vi "HumanExecute.vi"(8 "error in (no error)":errorcluster) -> (0 "error out":errorcluster)   [LabVIEW 2020]
doc: "Execute for Human\n\ninput:\n error in (cluster)\n\noutput:\n error out (cluster)"
uses:
  <vilib>/Rock Robotics/WPI/Joystick/XBox Buttons Indexer.ctl
  <vilib>/Rock Robotics/WPI/Joystick/XBox Axes Indexer.ctl
  Arm/ArmGamePiecePreset.ctl
  Arm/ArmPositionPreset.ctl
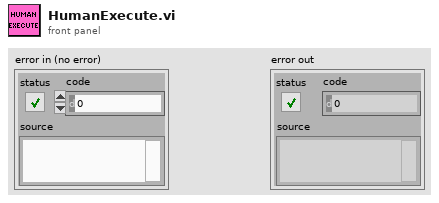
[diagram p1: front panel]
types:
  T1 = typedef "XBox Buttons Indexer.ctl" = enum16{"A", "B", "X", "Y", "Left Bumper", "Right Bumper", "Back", "Start", "Left Joystick", "Right Joystick"}
  T2 = typedef "XBox Axes Indexer.ctl" = enum16{"Left X", "Left Y", "Left Trigger", "Right Trigger", "Right X", "Right Y"}
  T3 = typedef "WPI_JoystickDevRef.ctl" = cluster{"Device":T4}
  T4 = typedef "WPI_JoystickDeviceEnum.ctl" = enum16{"USB 0", "USB 1", "USB 2", "USB 3", "USB 4", "USB 5"}
  T5 = typedef "ArmGamePiecePreset.ctl" = enum16{"Cube", "Cone"}
  T6 = typedef "ArmPositionPreset.ctl" = enum16{"Upper", "Lower", "Middle", "Shelf", "Floor"}
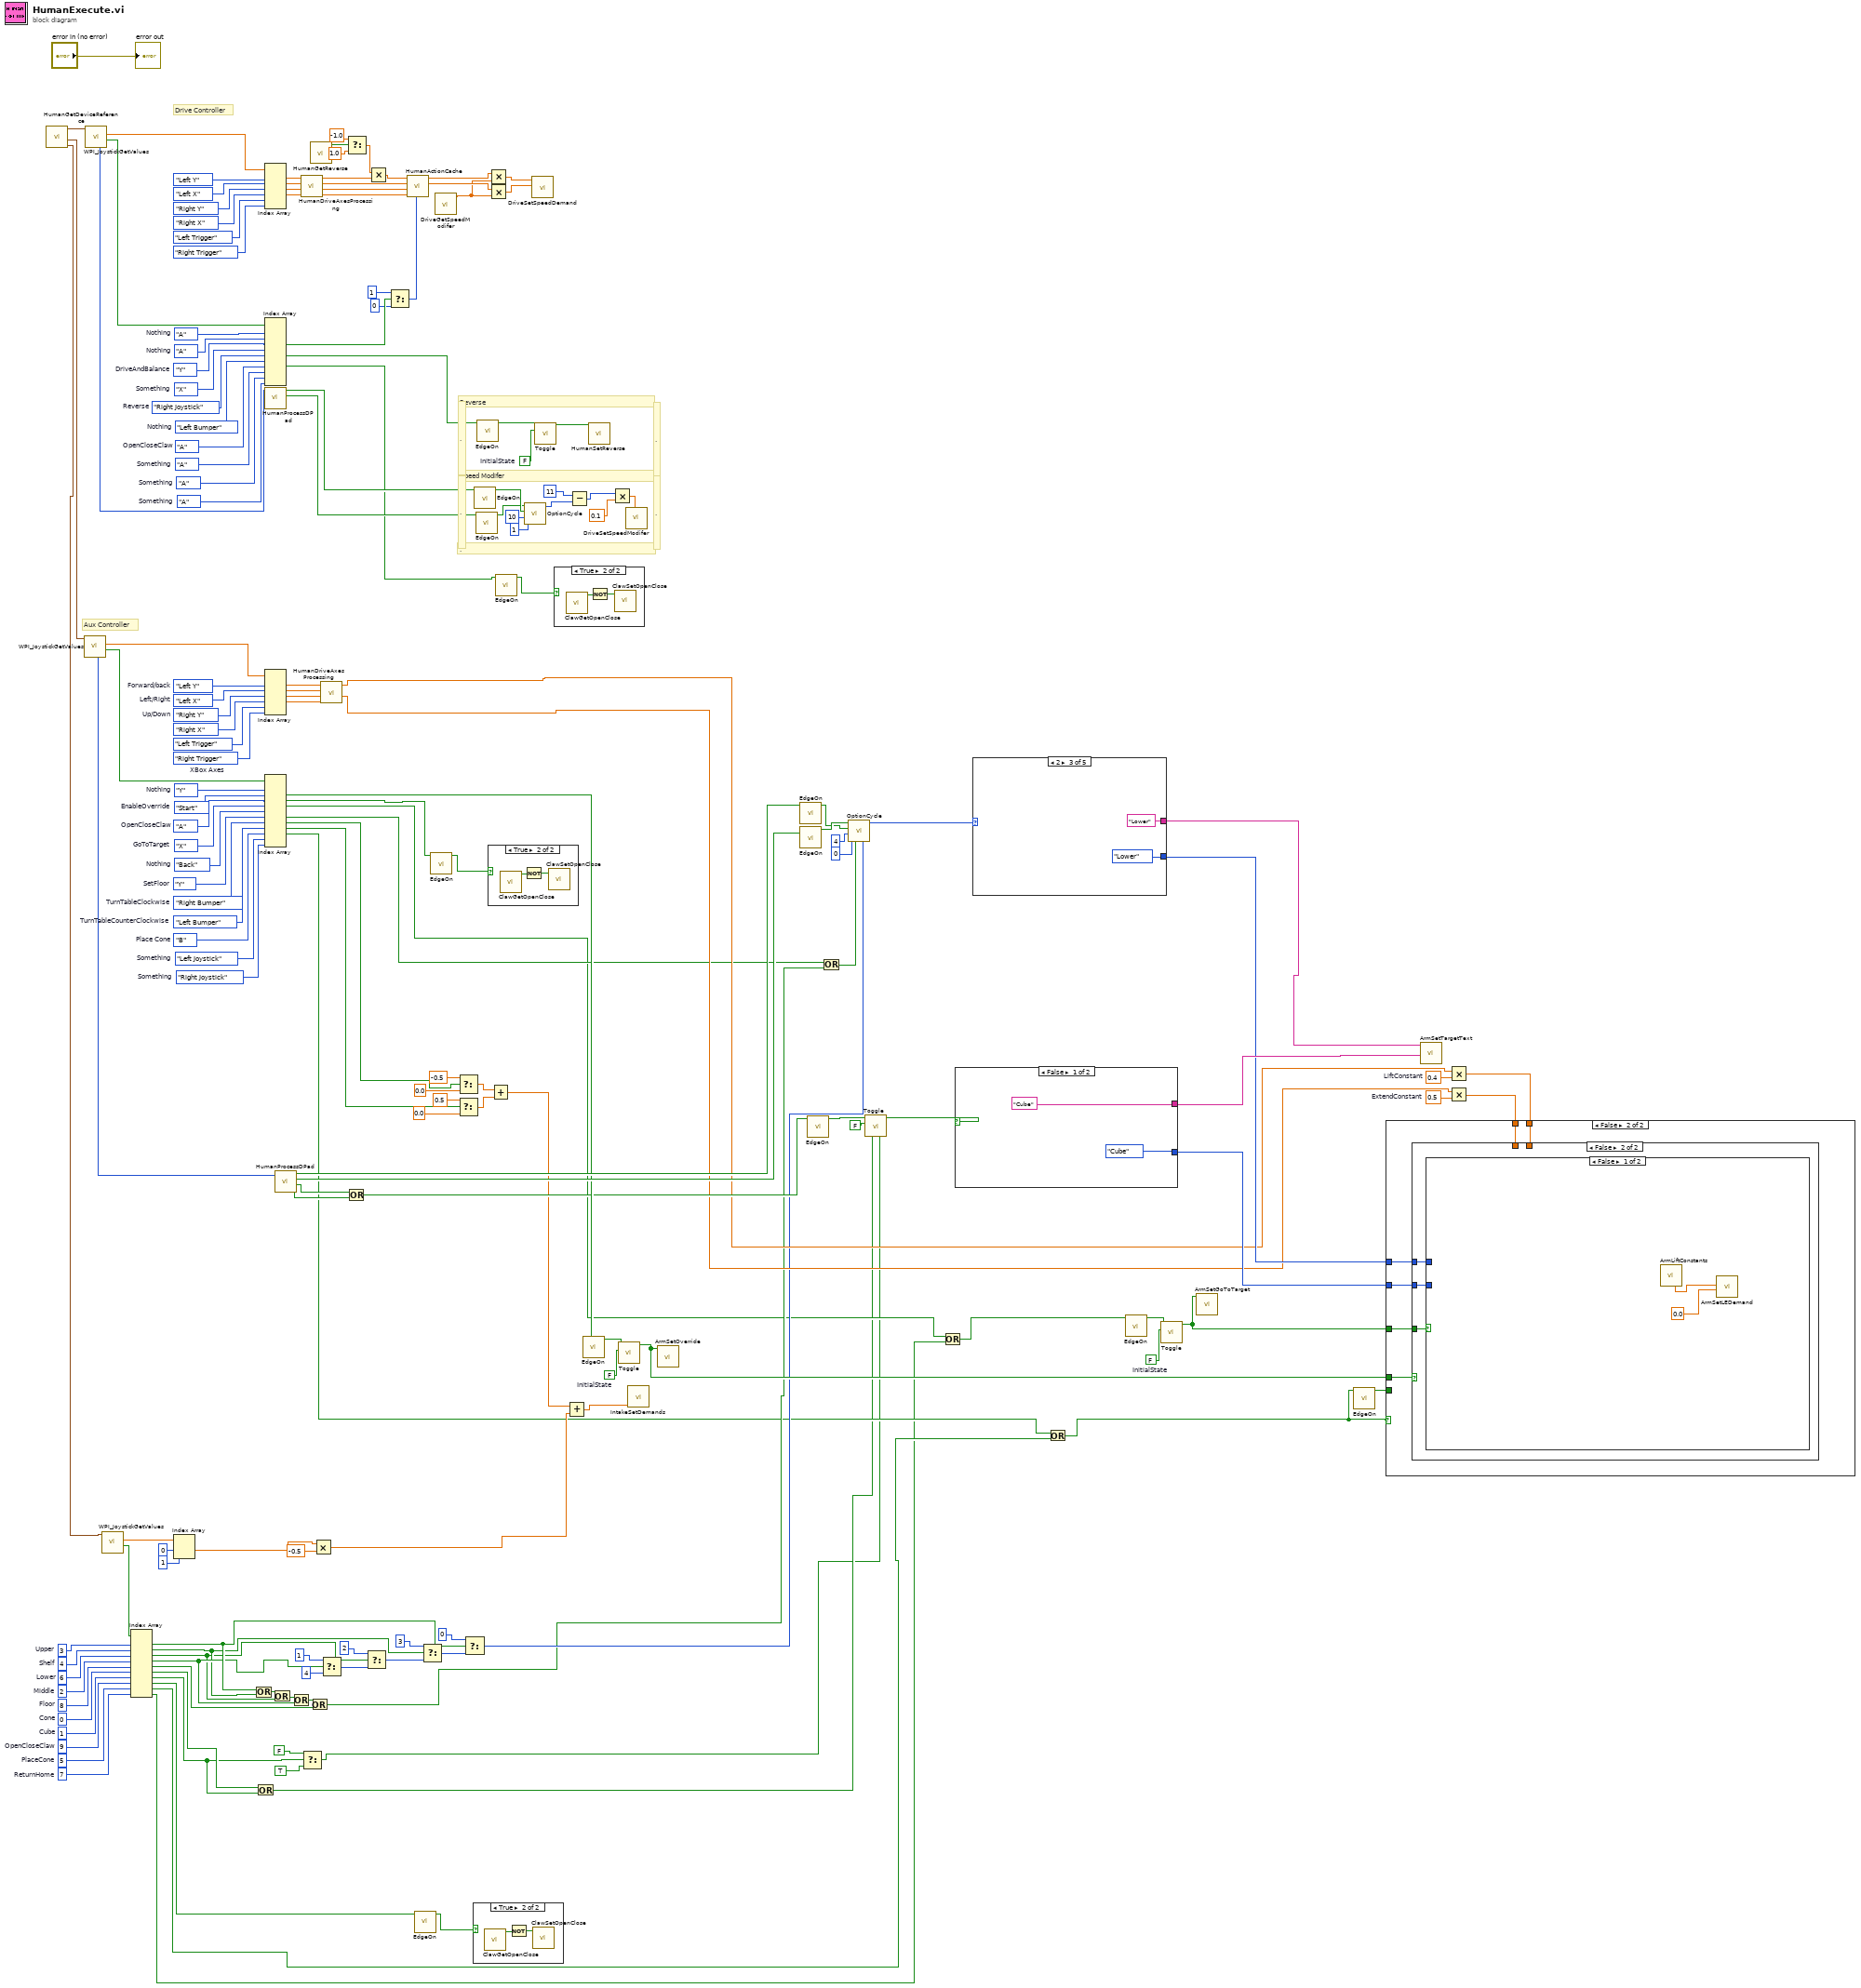
[diagram p0: block diagram]
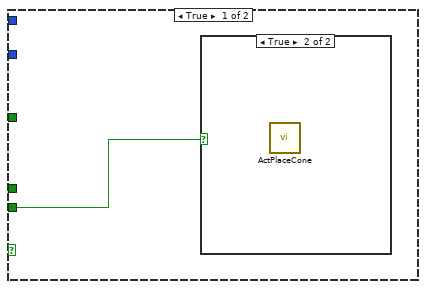
[diagram p2: hidden frame]
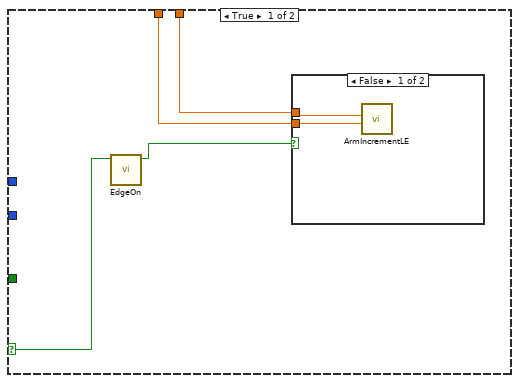
[diagram p4: hidden frame]
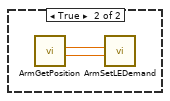
[diagram p5: hidden frame]
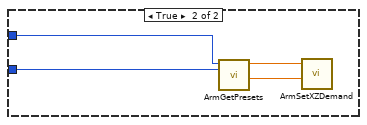
[diagram p6: hidden frame]
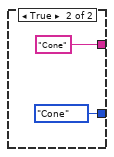
[diagram p10: hidden frame]
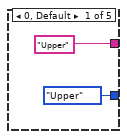
[diagram p11: hidden frame]
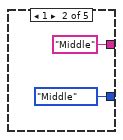
[diagram p12: hidden frame]
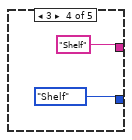
[diagram p13: hidden frame]
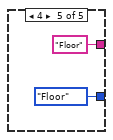
[diagram p14: hidden frame]
diagram:
  w15 = 0.4  # LiftConstant
  w16 = 0.5  # ExtendConstant
  w56 = 7  # ReturnHome
  w57 = 5  # PlaceCone
  w58 = 9  # OpenCloseClaw
  w59 = 1  # Cube
  w60 = 0  # Cone
  w61 = 8  # Floor
  w62 = 2  # Middle
  w63 = 6  # Lower
  w64 = 4  # Shelf
  w65 = 3  # Upper
  w93 = FALSE  # InitialState
  w95 = FALSE  # InitialState
  w121 = FALSE  # InitialState
  w130 = XBox_Buttons_Indexer."Right Joystick"  # Something
  w131 = XBox_Buttons_Indexer."Left Joystick"  # Something
  w132 = XBox_Buttons_Indexer."B"  # Place Cone
  w133 = XBox_Buttons_Indexer."Left Bumper"  # TurnTableCounterClockwise
  w134 = XBox_Buttons_Indexer."Right Bumper"  # TurnTableClockwise
  w135 = XBox_Buttons_Indexer."Y"  # SetFloor
  w136 = XBox_Buttons_Indexer."A"  # Something
  w137 = XBox_Buttons_Indexer."A"  # Something
  w138 = XBox_Buttons_Indexer."A"  # Something
  w139 = XBox_Buttons_Indexer."A"  # OpenCloseClaw
  w140 = XBox_Buttons_Indexer."Left Bumper"  # Nothing
  w157 = XBox_Buttons_Indexer."Back"  # Nothing
  w160 = XBox_Buttons_Indexer."X"  # GoToTarget
  w161 = XBox_Buttons_Indexer."A"  # OpenCloseClaw
  w162 = XBox_Buttons_Indexer."Start"  # EnableOverride
  w163 = XBox_Buttons_Indexer."Y"  # Nothing
  w153 = XBox_Axes_Indexer."Right Trigger"  # XBox Axes
  w156 = XBox_Axes_Indexer."Right Y"  # Up/Down
  w164 = XBox_Axes_Indexer."Left X"  # Left/Right
  w165 = XBox_Axes_Indexer."Left Y"  # Forward/back
  w168 = XBox_Buttons_Indexer."Right Joystick"  # Reverse
  w169 = XBox_Buttons_Indexer."X"  # Something
  w171 = XBox_Buttons_Indexer."Y"  # DriveAndBalance
  w172 = XBox_Buttons_Indexer."A"  # Nothing
  w173 = XBox_Buttons_Indexer."A"  # Nothing
  # "."
  # "Speed Modifer"
  # "."
  # "."
  # "."
  # "."
  # "Reverse"
  # "Drive Controller"
  # "Aux Controller"
  n1 = call "HumanGetDeviceReference.vi"() -> ("ButtonBoard"=w70:T3, "Aux Joy"=w175:T3, "Driver Joy"=w176:T3)  [unwired: 9 in]
  n2 = call <vilib>:"WPI_JoystickGetValues.vi"("JoystickDevRef"=w175) -> ("Buttons"=w158:bool[], "Axes"=w159:dbl[], "POVs"=w129:i16[])  [unwired: 6 in, 2 out]
  n3 = call <vilib>:"WPI_JoystickGetValues.vi"("JoystickDevRef"=w176) -> ("Buttons"=w174:bool[], "Axes"=w180:dbl[], "POVs"=w170:i16[])  [unwired: 6 in, 2 out]
  n4 = call <vilib>:"WPI_JoystickGetValues.vi"("JoystickDevRef"=w70) -> ("Buttons"=w69:bool[], "Axes"=w68:dbl[])  [unwired: 6 in, 3 out]
  n5 = Index Array "Index Array"(array=w69, index #1=w65, index #2=w64, index #3=w63, index #4=w62, index #5=w61, index #6=w60, index #7=w59, index #8=w58, index #9=w57, index #10=w56) -> (element #1=w42:bool, element #2=w40:bool, element #3=w3:bool, element #4=w41:bool, element #5=w39:bool, element #6=w33:bool, element #7=w32:bool, element #8=w34:bool, element #9=w7:bool, element #10=w4:bool)
  n6 = Index Array "Index Array"(array=w68, index #1=0 ("index"), index #2=1 ("index")) -> (element #1=w20:dbl)  [unwired: 1 out]
  n7 = Or(x=w42, y=w40) -> (x .or. y?=w45:bool)
  n8 = Or(x=w33, y=w32) -> (x .or. y?=w2:bool)
  n9 = Index Array(array=w180, index #1=XBox_Axes_Indexer."Left Y" ("XBox Axes"), index #2=XBox_Axes_Indexer."Left X" ("XBox Axes"), index #3=XBox_Axes_Indexer."Right Y" ("XBox Axes"), index #4=XBox_Axes_Indexer."Right X" ("XBox Axes"), index #5=XBox_Axes_Indexer."Left Trigger" ("XBox Axes"), index #6=XBox_Axes_Indexer."Right Trigger" ("XBox Axes")) -> (element #1=w148:dbl, element #2=w147:dbl, element #3=w146:dbl, element #4=w145:dbl)  [unwired: 2 out]
  n10 = Index Array(array=w174, index #1=w173, index #2=w172, index #3=w171, index #4=w169, index #5=w168, index #6=w140, index #7=w139, index #8=w138, index #9=w137, index #10=w136) -> (element #3=w141:bool, element #5=w119:bool, element #7=w37:bool)  [unwired: 7 out]
  n11 = call "HumanProcessDPad.vi"("POV"=w170) -> ("Down"=w107:bool, "Up"=w108:bool)  [unwired: 7 in, 2 out]
  n12 = Index Array(array=w159, index #1=w165, index #2=w164, index #3=w156, index #4=XBox_Axes_Indexer."Right X" ("XBox Axes"), index #5=XBox_Axes_Indexer."Left Trigger", index #6=w153) -> (element #1=w92:dbl, element #2=w91:dbl, element #3=w90:dbl, element #4=w89:dbl)  [unwired: 2 out]
  n13 = Index Array "Index Array"(array=w158, index #1=w163, index #2=w162, index #3=w161, index #4=w160, index #5=w157, index #6=w135, index #7=w134, index #8=w133, index #9=w132, index #10=w131, index #11=w130) -> (element #2=w72:bool, element #3=w38:bool, element #4=w6:bool, element #6=w13:bool, element #7=w81:bool, element #8=w82:bool, element #9=w9:bool)  [unwired: 4 out]
  n14 = Or(x=w45, y=w3) -> (x .or. y?=w44:bool)
  n15 = call "HumanProcessDPad.vi"("POV"=w129) -> ("Right"=w28:bool, "Left"=w29:bool, "Down"=w97:bool, "Up"=w98:bool)  [unwired: 7 in]
  n16 = Or(x=w44, y=w41) -> (x .or. y?=w43:bool)
  n17 = call "HumanDriveAxesProcessing.vi"("Right X"=w145, "Right Y"=w146, "Left X"=w147, "Left Y"=w148) -> ("Right X"=w142:dbl, "Right Y"=w143:dbl, "Left X"=w144:dbl, "Left Y"=w113:dbl)  [unwired: 4 in]
  n18 = Select(t=FALSE, s=w32, f=TRUE) -> (s? t:f=w1:bool)
  n19 = Or(x=w43, y=w39) -> (x .or. y?=w10:bool)
  n20 = call "HumanGetReverse.vi"() -> ("Reverse"=w117:bool)  [unwired: 11 in]
  n21 = Multiply(x=w20, y=-0.5) -> (x*y=w19:dbl)
  n22 = call "HumanDriveAxesProcessing.vi"("Right X"=w89, "Right Y"=w90, "Left X"=w91, "Left Y"=w92) -> ("Right Y"=w25:dbl, "Left Y"=w26:dbl)  [unwired: 4 in, 2 out]
  n23 = Select(t=1, s=w41, f=4) -> (s? t:f=w49:i32)
  n24 = Or(x=w29, y=w28) -> (x .or. y?=w27:bool)
  n25 = Select(t=-1.0, s=w117, f=1.0) -> (s? t:f=w114:dbl)
  n26 = Select(t=2, s=w3, f=w49) -> (s? t:f=w50:i32)
  n27 = Multiply(x=w114, y=w113) -> (x*y=w112:dbl)
  n28 = Select(t=1, s=w141, f=0) -> (s? t:f=w166:i32)
  n29 = call "HumanActionCache.vi"("State"=w166, "Right X"=w142, "Right Y"=w143, "Left X"=w144, "Left Y"=w112) -> ("RightMotorDemand"=w124:dbl, "LeftMotorDemand"=w125:dbl)  [unwired: 5 in]
  n30 = call "EdgeOn.vi"("Current State"=w34) -> ("Edge On Found"=w35:bool)  [unwired: 10 in]
  n31 = Select(t=3, s=w40, f=w50) -> (s? t:f=w47:i32)
  n32 = call "EdgeOn.vi"("Current State"=w38) -> ("Edge On Found"=w71:bool)  [unwired: 10 in]
  n33 = call "DriveGetSpeedModifer.vi"() -> ("SpeedModifer"=w120:dbl)  [unwired: 11 in]
  n34 = Select(t=-0.5, s=w81, f=0.0) -> (s? t:f=w88:dbl)
  n35 = Select(t=0.5, s=w82, f=0.0) -> (s? t:f=w87:dbl)
  n36 = Select(t=0, s=w42, f=w47) -> (s? t:f=w11:i32)
  n37 = case shown="True" w35 {
    frame False {
    }
    frame True {
      n38 = call "ClawGetOpenClose.vi"() -> ("Open?"=w182:bool)  [unwired: 11 in]
      n39 = Not(x=w182) -> (.not. x?=w181:bool)
      n40 = call "ClawSetOpenClose.vi"("Open?"=w181) -> ()  [unwired: 11 in]
    }
  }
  n41 = call "EdgeOn.vi"("Current State"=w108) -> ("Edge On Found"=w106:bool)  [unwired: 10 in]
  n42 = call "EdgeOn.vi"("Current State"=w107) -> ("Edge On Found"=w105:bool)  [unwired: 10 in]
  n43 = call "EdgeOn.vi"("Current State"=w119) -> ("Edge On Found"=w122:bool)  [unwired: 10 in]
  n44 = Multiply(x=w125, y=w120) -> (x*y=w127:dbl)
  n45 = Multiply(x=w124, y=w120) -> (x*y=w126:dbl)
  n46 = case shown="True" w71 {
    frame False {
    }
    frame True {
      n47 = call "ClawGetOpenClose.vi"() -> ("Open?"=w184:bool)  [unwired: 11 in]
      n48 = Not(x=w184) -> (.not. x?=w183:bool)
      n49 = call "ClawSetOpenClose.vi"("Open?"=w183) -> ()  [unwired: 11 in]
    }
  }
  n50 = Add(x=w88, y=w87) -> (x+y=w22:dbl)
  n51 = call "EdgeOn.vi"("Current State"=w37) -> ("Edge On Found"=w36:bool)  [unwired: 10 in]
  n52 = call "OptionCycle.vi"("MinValue"=1, "MaxValue"=10, "BackwardsInput"=w106, "ForwardInput"=w105) -> ("CycleNum"=w111:i32)  [unwired: 7 in]
  n53 = call "DriveSetSpeedDemand.vi"("RSpeedDemand (ft/s)"=w126, "LSpeedDemand (ft/s)"=w127) -> ()  [unwired: 10 in]
  n54 = call "Toggle.vi"("InitialState"=w121, "FlashInput"=w122) -> ("Toggled"=w118:bool)  [unwired: 9 in]
  n55 = case shown="True" w36 {
    frame False {
    }
    frame True {
      n56 = call "ClawGetOpenClose.vi"() -> ("Open?"=w186:bool)  [unwired: 11 in]
      n57 = Not(x=w186) -> (.not. x?=w185:bool)
      n58 = call "ClawSetOpenClose.vi"("Open?"=w185) -> ()  [unwired: 11 in]
    }
  }
  n59 = Add(x=w22, y=w19) -> (x+y=w23:dbl)
  n60 = Subtract(x=11, y=w111) -> (x-y=w109:i32)
  n61 = call "EdgeOn.vi"("Current State"=w72) -> ("Edge On Found"=w96:bool)  [unwired: 10 in]
  n62 = call "HumanSetReverse.vi"("Reverse"=w118) -> ()  [unwired: 11 in]
  n63 = Multiply(x=w109, y=0.1) -> (x*y=w123:dbl)
  n64 = call "Toggle.vi"("InitialState"=w95, "FlashInput"=w96) -> ("Toggled"=w24:bool)  [unwired: 9 in]
  n65 = call "DriveSetSpeedModifer.vi"("SpeedModifer"=w123) -> ()  [unwired: 11 in]
  n66 = call "IntakeSetDemands.vi"("turntableDemand"=w23) -> ()  [unwired: 11 in]
  n67 = call "ArmSetOverride.vi"("Override"=w24) -> ()  [unwired: 11 in]
  n68 = call "EdgeOn.vi"("Current State"=w98) -> ("Edge On Found"=w54:bool)  [unwired: 10 in]
  n69 = call "EdgeOn.vi"("Current State"=w97) -> ("Edge On Found"=w55:bool)  [unwired: 10 in]
  n70 = call "EdgeOn.vi"("Current State"=w27) -> ("Edge On Found"=w99:bool)  [unwired: 10 in]
  n71 = Or(x=w13, y=w10) -> (x .or. y?=w12:bool)
  n72 = call "OptionCycle.vi"("ValuetoSet"=w11, "SetValue"=w12, "MinValue"=0, "MaxValue"=4, "BackwardsInput"=w54, "ForwardInput"=w55) -> ("CycleNum"=w104:i32)  [unwired: 5 in]
  n73 = call "Toggle.vi"("State to Set"=w1, "SetState"=w2, "InitialState"=FALSE, "FlashInput"=w99) -> ("Toggled"=w101:bool)  [unwired: 7 in]
  n74 = Or(x=w6, y=w4) -> (x .or. y?=w5:bool)
  n75 = case shown="False" w101 {
    tunnel: ["Cube" "Cone"] -> w75
    tunnel: [ArmGamePiecePreset."Cube" ("Game Piece") ArmGamePiecePreset."Cone" ("Game Piece")] -> w74
    frame False {
    }
    frame True {
    }
  }
  n76 = case shown="2" w104 {
    tunnel: ["Upper" "Middle" "Lower" "Shelf" "Floor"] -> w76
    tunnel: [ArmPositionPreset."Upper" ("Position") ArmPositionPreset."Middle" ("Position") ArmPositionPreset."Lower" ("Position") ArmPositionPreset."Shelf" ("Position") ArmPositionPreset."Floor" ("Position")] -> w73
    frame 0, Default {
    }
    frame 1 {
    }
    frame 2 {
    }
    frame 3 {
    }
    frame 4 {
    }
  }
  n77 = Or(x=w9, y=w7) -> (x .or. y?=w8:bool)
  n78 = call "EdgeOn.vi"("Current State"=w5) -> ("Edge On Found"=w94:bool)  [unwired: 10 in]
  n79 = call "Toggle.vi"("InitialState"=w93, "FlashInput"=w94) -> ("Toggled"=w78:bool)  [unwired: 9 in]
  n80 = call "ArmSetGoToTarget.vi"("HeadingToTarget"=w78) -> ()  [unwired: 11 in]
  n81 = call "EdgeOn.vi"("Current State"=w8) -> ("Edge On Found"=w14:bool)  [unwired: 10 in]
  n82 = call "ArmSetTargetText.vi"("TargetGamePiece"=w75, "TargetArmPosition"=w76) -> ()  [unwired: 10 in]
  n83 = Multiply(x=w26, y=w15) -> (x*y=w18:dbl)
  n84 = Multiply(x=w25, y=w16) -> (x*y=w17:dbl)
  n85 = case shown="False" w8 {
    tunnel: w24 -> [_ w207]
    tunnel: w78 -> [_ w206]
    tunnel: w18 -> [_ w205]
    tunnel: w17 -> [_ w204]
    tunnel: w74 -> [_ w203]
    tunnel: w73 -> [_ w202]
    tunnel: w14 -> [w201 _]
    frame True {
      n86 = case shown="True" w201 {
        frame False {
        }
        frame True {
          n87 = call "ActPlaceCone.vi"() -> ()  [unwired: 11 in, 1 out]
        }
      }
    }
    frame False {
      n88 = case shown="False" w207 {
        selector: w207 -> [w211 _]
        tunnel: w206 -> [_ w218]
        tunnel: w205 -> [w208 _]
        tunnel: w204 -> [w209 _]
        tunnel: w203 -> [_ w217]
        tunnel: w202 -> [_ w216]
        frame True {
          n89 = call "EdgeOn.vi"("Current State"=w211) -> ("Edge On Found"=w210:bool)  [unwired: 10 in]
          n90 = case shown="False" w210 {
            tunnel: w209 -> [w213 _]
            tunnel: w208 -> [w212 _]
            frame False {
              n91 = call "ArmIncrementLE.vi"("AddE"=w213, "AddL"=w212) -> ()  [unwired: 10 in]
            }
            frame True {
              n92 = call "ArmGetPosition.vi"() -> ("ExtendPostion"=w214:dbl, "LiftPostion"=w215:dbl)  [unwired: 10 in]
              n93 = call "ArmSetLEDemand.vi"("SetExtendPositonDemand(in)"=w214, "SetLIftPostionDemand(d)"=w215) -> ()  [unwired: 10 in]
            }
          }
        }
        frame False {
          n94 = case shown="False" w218 {
            tunnel: w217 -> [_ w222]
            tunnel: w216 -> [_ w221]
            frame False {
              n95 = call "ArmLiftConstants.vi"() -> ("Default Angle"=w219:dbl)  [unwired: 8 in, 3 out]
              n96 = call "ArmSetLEDemand.vi"("SetExtendPositonDemand(in)"=0.0, "SetLIftPostionDemand(d)"=w219) -> ()  [unwired: 10 in]
            }
            frame True {
              n97 = call "ArmGetPresets.vi"("Game Piece"=w222, "Position"=w221) -> ("z"=w223:dbl, "x"=w224:dbl)  [unwired: 8 in]
              n98 = call "ArmSetXZDemand.vi"("SetZ"=w223, "SetX"=w224) -> ()  [unwired: 10 in]
            }
          }
        }
      }
    }
  }
  "error out" <- "error in (no error)"
